vi "Modbus to Char.vi"(10 "Register In":u16) -> (2 "Unsigned Char":string)   [LabVIEW 2024, in "Bronkhorst Flexi-Flow ModbusTCP API.lvlib"]
uses:
  Bronkhorst Flexi-Flow ModbusTCP API.lvlib
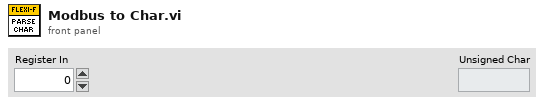
[diagram p1: front panel]
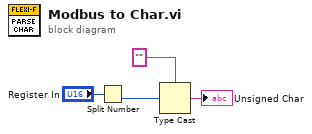
[diagram p0: block diagram]
diagram:
  n1 = Split Number(x="Register In") -> (lo(x)=w3:u8)  [unwired: 1 out]
  n2 = Type Cast(type="", x=w3) -> (*(type *) &x=→"Unsigned Char":string)
